vi "Update ClockID.vi"(8 "error in (no error)":errorcluster, 10 "ClockID":u8, 11 "CIF_NIChn_FifoCAN in":refnum<class "CIF_NIChn_FifoCAN.lvclass">) -> (0 "error out":errorcluster, 3 "CIF_NIChn_FifoCAN out":refnum<class "CIF_NIChn_FifoCAN.lvclass">)   [LabVIEW 2021, in "CIF_NIChn_FifoCAN.lvclass"]
uses:
  CIF_NIChn_FifoCAN.lvclass
  CIF_NIChn_FifoCAN.lvclass/CIF_NIChn_FifoCAN.ctl
  ChannelCommon/CIFFIFO/CIFfifo.lvclass
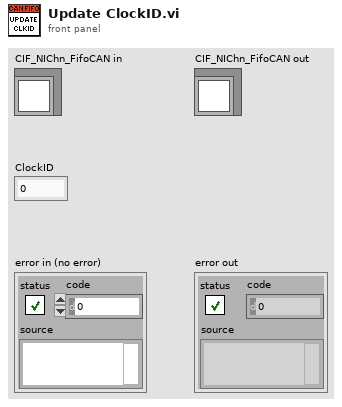
[diagram p1: front panel]
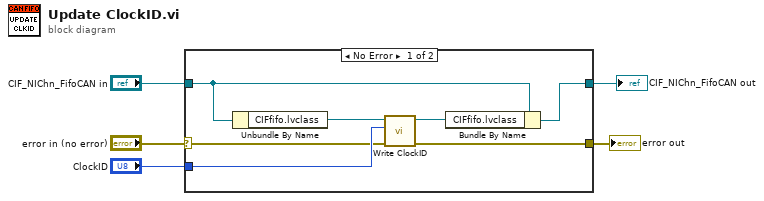
[diagram p0: block diagram]
diagram:
  n1 = case shown="No Error" "error in (no error)" {
    selector: "error in (no error)" -> [w7 w14]
    tunnel: [w6 w14] -> w4
    tunnel: [w9 w13] -> w2
    tunnel: "CIF_NIChn_FifoCAN in" -> [w11 w13]
    tunnel: "ClockID" -> [w8 _]
    frame No Error {
      n2 = Unbundle By Name(w11) -> ("CIFfifo.lvclass"=w12:refnum<class "CIFfifo.lvclass">)
      n3 = call "Write ClockID.vi"("error in (no error)"=w7, "ClockID"=w8, "CIFfifo in"=w12) -> ("error out"=w6:errorcluster, "CIFfifo out"=w10:refnum<class "CIFfifo.lvclass">)  [unwired: 7 in]
      n4 = Bundle By Name(cluster=w11, "CIFfifo.lvclass"=w10) -> (w9:refnum<class "CIF_NIChn_FifoCAN.lvclass">)
    }
    frame Error {
    }
  }
  "error out" <- w4
  "CIF_NIChn_FifoCAN out" <- w2
